vi "PS Control Status String.vi"(10 "VI Name":string="PS Control.vi") -> (0 "error out":errorcluster, 1 "Status String":string)   [LabVIEW 2025]
doc: "Author: Scott Hannahs <sth@magnet.fsu.edu>\n\nThis software is licensed for use under the “MIT License\"\nCopyright (c) 2025 Scott Hannahs, sth@sth@magnet.sthnet.net\n\nPermission is hereby granted, free of charge, to any person obtaining a copy of this software and associated documentation files (the \"Software\"), to deal in the Software without restriction, including without limitation the rights to use, copy, modify, merge, publish, distribute, sublicense, and/or sell copies of the Software, and to permit persons to whom the Software is furnished to do so, subject to the following conditions: The above copyright notice and this permission notice shall be included in all copies or substantial portions of the Software.\n\nTHE SOFTWARE IS PROVIDED \"AS IS\", WITHOUT WARRANTY OF ANY KIND, EXPRESS OR IMPLIED, INCLUDING BUT NOT LIMITED TO THE WARRANTIES OF MERCHANTABILITY, FITNESS FOR A PARTICULAR PURPOSE AND NONINFRINGEMENT. IN NO EVENT SHALL THE AUTHORS OR COPYRIGHT HOLDERS BE LIABLE FOR ANY CLAIM, DAMAGES OR OTHER LIABILITY, WHETHER IN AN ACTION OF CONTRACT, TORT OR OTHERWISE, ARISING FROM, OUT OF OR IN CONNECTION WITH THE SOFTWARE OR THE USE OR OTHER DEALINGS IN THE SOFTWARE."
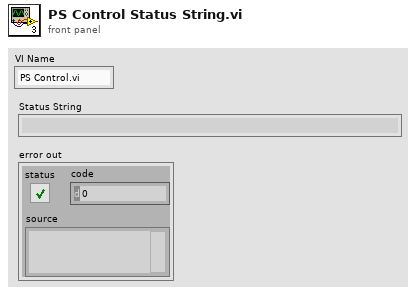
[diagram p1: front panel]
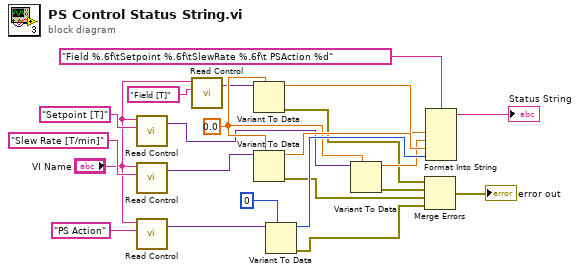
[diagram p0: block diagram]
diagram:
  w9 = 0.0
  n1 = call "Read Control.vi"("VI Name"="VI Name", "Control Name"="Setpoint [T]") -> ("Value"=w7:variant)  [unwired: 3 in, 1 out]
  n2 = call "Read Control.vi"("VI Name"="VI Name", "Control Name"="Slew Rate [T/min]") -> ("Value"=w6:variant)  [unwired: 3 in, 1 out]
  n3 = call "Read Control.vi"("VI Name"="VI Name", "Control Name"="PS Action") -> ("Value"=w10:variant)  [unwired: 3 in, 1 out]
  n4 = call "Read Control.vi"("VI Name"="VI Name", "Control Name"="Field [T]") -> ("Value"=w8:variant)  [unwired: 3 in, 1 out]
  n5 = Variant To Data(type=w9, Variant=w8) -> (data=w17:dbl, error out=w12:errorcluster)  [unwired: 1 in]
  n6 = Variant To Data(type=w9, Variant=w6) -> (data=w19:dbl, error out=w14:errorcluster)  [unwired: 1 in]
  n7 = Variant To Data(type=0, Variant=w10) -> (data=w20:i32, error out=w15:errorcluster)  [unwired: 1 in]
  n8 = Variant To Data(type=w9, Variant=w7) -> (data=w18:dbl, error out=w13:errorcluster)  [unwired: 1 in]
  n9 = Merge Errors(w12, w13, w14, w15) -> (→"error out":errorcluster)
  n10 = Format Into String(format string="Field %.6f\tSetpoint %.6f\tSlewRate %.6f\t PSAction %d", w17, w18, w19, w20) -> (resulting string=→"Status String":string)  [unwired: 2 in, 1 out]
